vi "zadanie_8_spirala.vi"() -> ()   [LabVIEW 2024]
panel:
  in  "Scale":dbl
  out "XY Graph":cluster{dbl[], dbl[]}(graph)
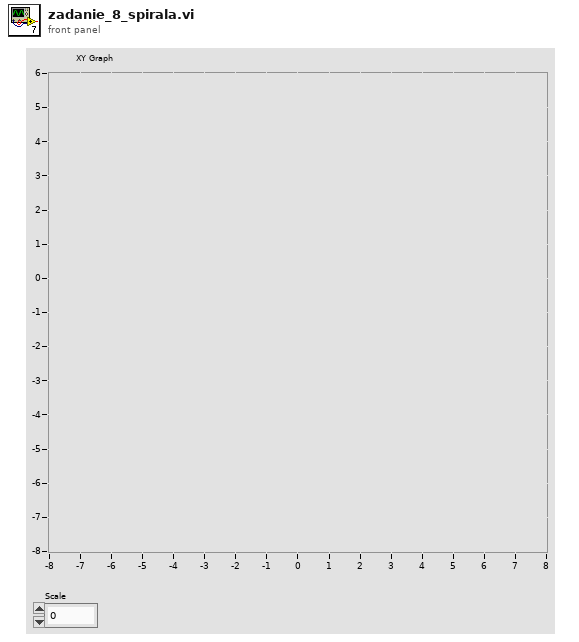
[diagram p1: front panel]
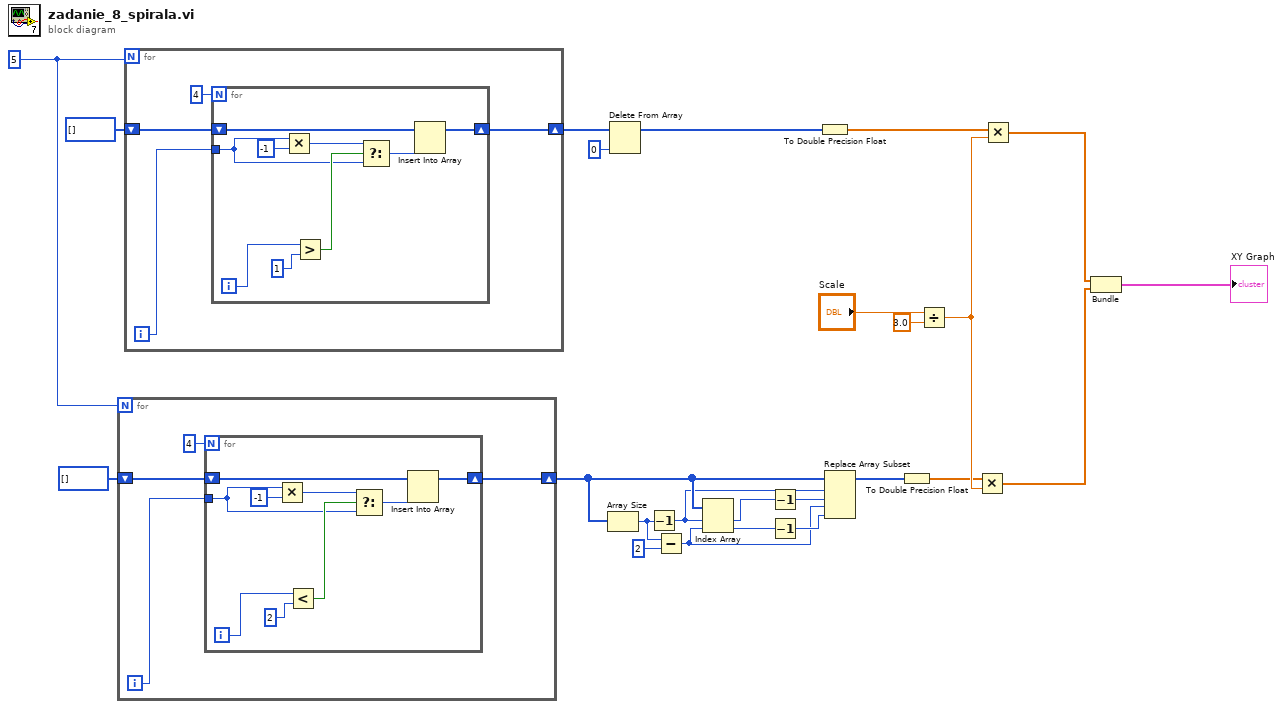
[diagram p0: block diagram]
diagram:
  w6 = 5
  n1 = for {
    N: w6 -> [_]
    shift-right: [w26] -> w11
    shift-left: i32[] [] -> [w25]
    i -> [w28]
    n2 = for {
      N: 4 -> [_]
      tunnel: w28 -> [w30]
      shift-right: [w37] -> w26
      shift-left: w25 -> [w36]
      i -> [w35]
      n3 = Multiply(x=w30, y=-1) -> (x*y=w31:i32)
      n4 = Less?(x=w35, y=2) -> (x < y?=w33:bool)
      n5 = Select(t=w31, s=w33, f=w30) -> (s? t:f=w29:i32)
      n6 = Insert Into Array(array=w36, new element=w29) -> (w37:i32[])  [unwired: 1 in]
    }
  }
  n7 = for {
    N: w6 -> [_]
    shift-right: [w39] -> w22
    shift-left: i32[] [] -> [w38]
    i -> [w41]
    n8 = for {
      N: 4 -> [_]
      tunnel: w41 -> [w43]
      shift-right: [w50] -> w39
      shift-left: w38 -> [w49]
      i -> [w48]
      n9 = Multiply(x=w43, y=-1) -> (x*y=w44:i32)
      n10 = Greater?(x=w48, y=1) -> (0:w46:bool)
      n11 = Select(t=w44, s=w46, f=w43) -> (s? t:f=w42:i32)
      n12 = Insert Into Array(array=w49, new element=w42) -> (w50:i32[])  [unwired: 1 in]
    }
  }
  n13 = Array Size(array=w11) -> (size(s)=w10:i32)
  n14 = Delete From Array(array=w22, index=0) -> (array with subset deleted=w17:i32[])  [unwired: 1 in, 1 out]
  n15 = Decrement(x=w10) -> (x-1=w8:i32)
  n16 = Subtract(x=w10, y=2) -> (x-y=w7:i32)
  n17 = Index Array(array=w11, index #1=w8, index #2=w7) -> (element #1=w15:i32, element #2=w13:i32)
  n18 = Decrement(x=w15) -> (x-1=w14:i32)
  n19 = Decrement(x=w13) -> (x-1=w12:i32)
  n20 = To Double Precision Float(number=w17) -> (double precision float=w3:dbl[])
  n21 = Replace Array Subset(array=w11, new element #1=w14, index #1=w8, new element #2=w12, index #2=w7) -> (w16:i32[])
  n22 = To Double Precision Float(number=w16) -> (double precision float=w2:dbl[])
  n23 = Divide(x="Scale", y=3.0) -> (x/y=w5:dbl)
  n24 = Multiply(x=w2, y=w5) -> (x*y=w18:dbl[])
  n25 = Multiply(x=w3, y=w5) -> (x*y=w19:dbl[])
  n26 = Bundle(w19, w18) -> (→"XY Graph":cluster{dbl[], dbl[]})  [unwired: 1 in]
